vi "Configure Acquisition.vi"(0 "device session in":refnum<class "Device Session.lvclass">, 1 "pretrigger samples":u64, 2 "number of records is finite (T)":bool=TRUE, 5 "number of records":u64=1, 7 "number of samples":u64=1000, 9 "channels to store":u32[](array[numeric]), 11 "error in":errorcluster, 12 "additional configuration":T3={"record padding (samples)"=0, "require finite records to fit in memory"=TRUE, "timestamps per record"=1, "status fifo depth (records)"=10000}, 13 "Chan#":T2=enum."1") -> (4 "device session out":refnum<class "Device Session.lvclass">, 6 "actual channels stored":bool[](array[boolean]), 8 "TrigCount":u32[](array[numeric]), 10 "TrigCfg Array":T1(array[cluster]), 15 "error out":errorcluster)   [LabVIEW 2021, in "Device Session.lvclass"]
doc: "Configures the acquisition. You can specify which channels to acquire from, how many records to acquire, and how many samples to acquire. You must run this VI before running the <B>Initiate</B> VI.\n\n<B>Input Parameters</B>\n\n<B>device session in</B> is a reference to the Device Session object, which contains a session to each instrument design library used in this sample project. This parameter is obtained from the 'Open Session' VI.\n\n<B>number of records is finite (T)</B> specifies whether to acquire a finite number of records, or to acquire records continuously.\n\n<B>pretrigger samples</B> specifies, for every record, the minimum number of samples that must be stored from the time period immediately before the Reference Trigger occurred.\n\n<B>number of records</B> specifies the number of records to acquire. The default value is 1.\n\n<B>number of samples</B> specifies the number of samples to acquire. The default value is 1000.\n\n<B>channels to store</B> specifies the channels to store in memory. By default, only the channels configured using the 'Configure Channel' VI are stored.\n\n<B>additional configuration</B> specifies additional advanced configurations.\n\n<B>additional configuration.record padding (samples)</B> specifies additional padding to allocate for a record. This parameter can be useful in combination with adjusting the Reference Trigger position. The default value is 0.\n\n<B>additional configuration.require finite records to fit in memory</B> specifies that the requested number of records and samples must fit into memory for finite acquisitions. This parameter ensures that requested data cannot be overwritten for finite acquisitions. The default is TRUE.\n\n<B>additional configuration.timestamps per record</B> specifies the number of timestamp values the FPGA captures for each record. This value must match the number of timestamps per record provided to the Write VI of the Multirecord Acquisition FPGA library. The default value is 0.\n\n<B>additional configuration.status fifo depth (records)</B> Sets the depth of the record status DMA FIFO. The Status FIFO reports information about the current state of the acquisition to the host.\nEnsure that the Status FIFO is deep enough for the rate at which the host consumes this FIFO. If the Status FIFO is full, memory writes are delayed. Eventually, this can cause the Write FIFO to fill up and overflow. The host consumes the entire Status FIFO each time you fetch a record or query acquisition status. The value is specified in units of records. The default value is 10,000 records.\n\n<B>error in</B> describes error conditions that occur before this node runs. This input provides standard 'error in' functionality.\n\n<B>Output Parameters</B>\n\n<B>device session out</B> passes a reference to the session to the next VI.\n\n<B>actual channels stored</B> returns the number of channels stored as a power of two.\n\n<B>error out</B> contains error information. This output provides standard 'error out' functionality."
uses:
  Device Session.lvclass
  <instrlib>/_niInstr/Multirecord Acquisition/Interface/v1/Host/Public/Additional Acquisition Configuration.ctl
  Enums/Channel Numbers.ctl
  Device Session.lvclass/Device Session.ctl
  <vilib>/Utility/error.llb/Error Cluster From Error Code.vi
  <vilib>/rvi/errors/niLvFpgaAdjustHostInterfaceError.vi
  <vilib>/rvi/interface/nirviReadWriteControl/nirviReadWriteControl.xnode
  FPGA Refnum.ctl
  <instrlib>/_niInstr/Multirecord Acquisition/Interface/v1/Host/niInstr Multirecord Acquisition v1 Host.lvclass
  <vilib>/rvi/interface/Simulation/niFpgaSimulationCallBeginRW.vi
  NiFpgaLv.dll
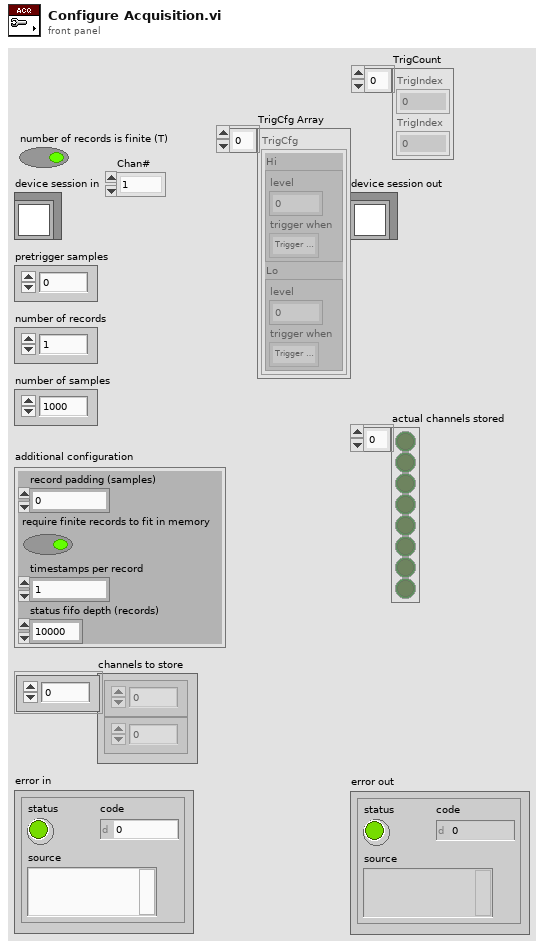
[diagram p1: front panel]
types:
  T1 = cluster{"Hi":cluster{"level":fxp<+/-,18,5>, "trigger when":enum8{"Trigger Above", "Trigger Below"}}, "Lo":cluster{"level":fxp<+/-,18,5>, "trigger when":enum8{"Trigger Above", "Trigger Below"}}}[]
  T2 = typedef "Channel Numbers.ctl" = enum16{"0", "1", "2", "3", "4", "5", "6", "7"}
  T3 = typedef "niInstr Multirecord Acquisition v1 Host.lvclass/Additional Acquisition Configuration.ctl" = cluster{"record padding (samples)":u64, "require finite records to fit in memory":bool, "timestamps per record":u32, "status fifo depth (records)":u32}
  T4 = typedef "Device Session.lvclass/Device Session Object.ctl" = cluster{"fpga reference":T5, "reg bus":refnum<class "niInstr FIFO Register Bus v1 Host.lvclass">, "subsystem map":refnum<class "niInstr Subsystem Map v1 Host.lvclass">, "cal data":refnum<class "niHSAI Cal Data v1 Host.lvclass">, "config":refnum<class "niHSAI Group A Config v1 Host.lvclass">, "acquisition 0":refnum<class "niInstr Multirecord Acquisition v1 Host.lvclass">, "acquisition 1":refnum<class "niInstr Multirecord Acquisition v1 Host.lvclass">, "acquisition 2":refnum<class "niInstr Multirecord Acquisition v1 Host.lvclass">, "acquisition 3":refnum<class "niInstr Multirecord Acquisition v1 Host.lvclass">, "acquisition 4":refnum<class "niInstr Multirecord Acquisition v1 Host.lvclass">, "acquisition 5":refnum<class "niInstr Multirecord Acquisition v1 Host.lvclass">, "acquisition 6":refnum<class "niInstr Multirecord Acquisition v1 Host.lvclass">, "acquisition 7":refnum<class "niInstr Multirecord Acquisition v1 Host.lvclass">, "number of selected acq channels":u8, "selected acq channels":bool[], "number of channels":u32, "configured channels":bool[], "acq configuration":cluster{"number of samples":u64, "number of records":u64, "pretrigger samples":u64}, "actual channel configuration":T6[], "sample clock rate (Hz)":dbl, "scaling coefficients":T10[]}
  T5 = typedef "Device Session.lvclass/FPGA Refnum.ctl" = refnum<k20>
  T6 = typedef "niHSAI Types v1 Host.lvlib/Channel Configuration.ctl" = cluster{"channel":u32, "coupling":T7, "impedance":T8, "bandwidth":T9, "vertical range":dbl, "vertical offset":dbl}
  T7 = typedef "niHSAI Types v1 Host.lvlib/Coupling.ctl" = enum8{"Default", "DC", "AC"}
  T8 = typedef "niHSAI Types v1 Host.lvlib/Impedance.ctl" = enum8{"Default", "1 mega ohm", "50 ohm"}
  T9 = typedef "niHSAI Types v1 Host.lvlib/Bandwidth.ctl" = enum8{"Default", "Full Bandwidth", "Anti-alias Filter", "150 MHz"}
  T10 = typedef "niInstr Multirecord Acquisition v1 Host.lvclass/Scaling Coefficient.ctl" = cluster{"gain":dbl, "offset":dbl}
  T11 = cluster{"Hi":cluster{"level":fxp<+/-,18,5>, "trigger when":enum8{"Trigger Above", "Trigger Below"}}, "Lo":cluster{"level":fxp<+/-,18,5>, "trigger when":enum8{"Trigger Above", "Trigger Below"}}}
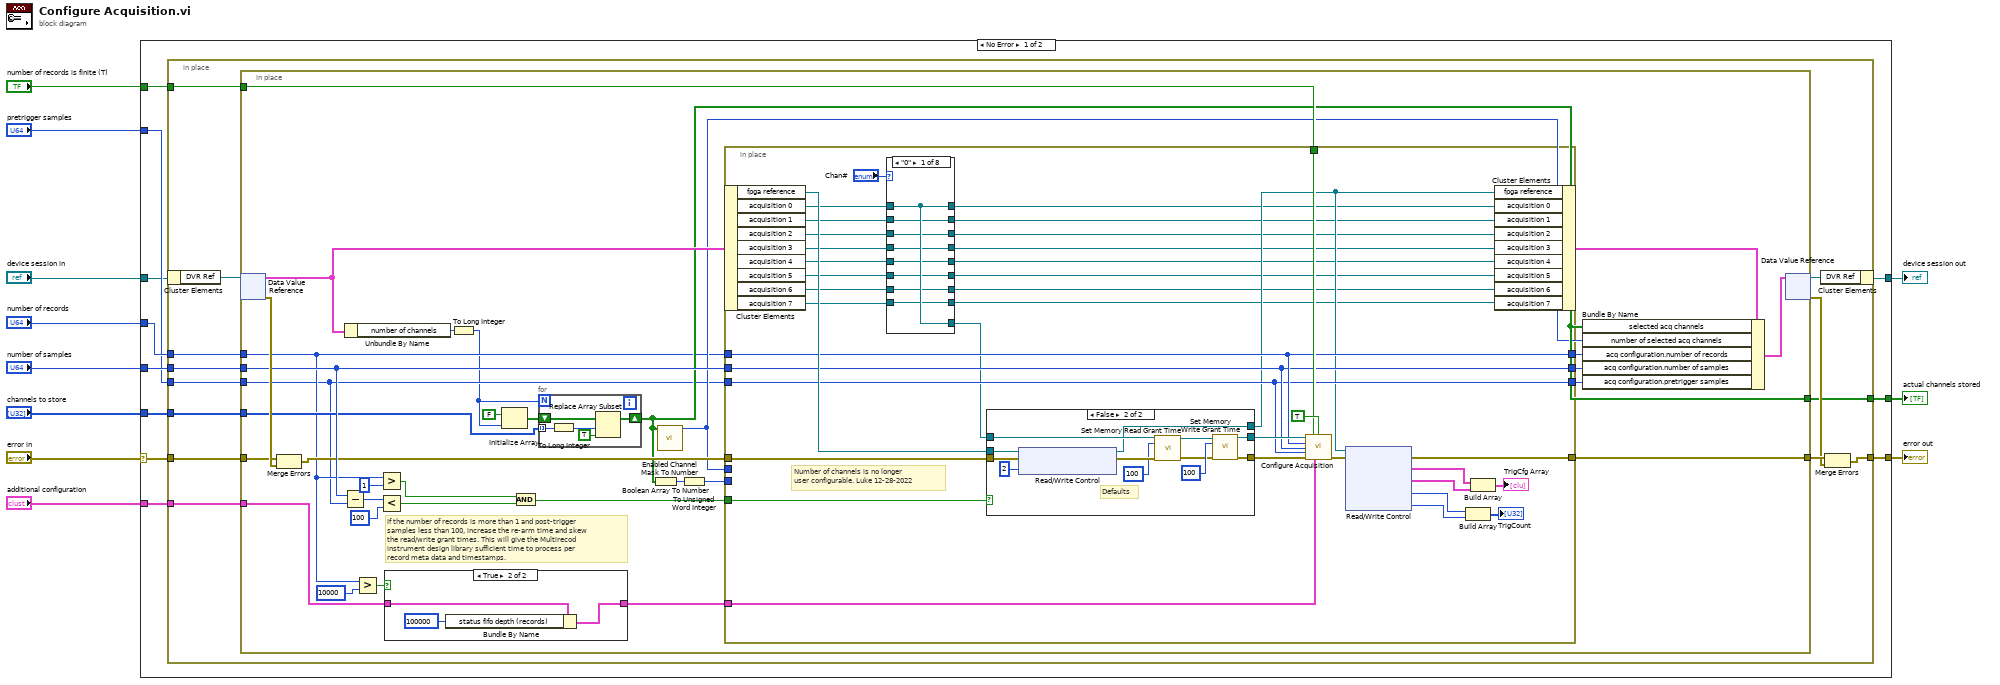
[diagram p0: block diagram]
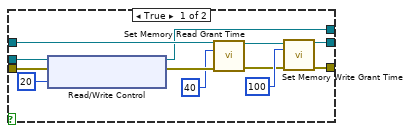
[diagram p9: hidden frame]
diagram:
  n1 = case shown="No Error" "error in" {
    selector: "error in" -> [w22 w205]
    tunnel: [w14 w205] -> w10
    tunnel: "device session in" -> [w12 w204]
    tunnel: [w13 w204] -> w8
    tunnel: "number of records" -> [w21 _]
    tunnel: "number of samples" -> [w20 _]
    tunnel: "channels to store" -> [w19 _]
    tunnel: [w18 _] -> w4
    tunnel: "pretrigger samples" -> [w17 _]
    tunnel: "additional configuration" -> [w16 _]
    tunnel: "number of records is finite (T)" -> [w15 _]
    frame No Error {
      n2 = in-place {
        in-place-border: w22 -> [w35]
        in-place-border: w21 -> [w34]
        in-place-border: w20 -> [w33]
        in-place-border: w19 -> [w30]
        in-place-border: [w29] -> w18
        in-place-border: w17 -> [w28]
        in-place-border: w16 -> [w27]
        in-place-border: w15 -> [w26]
        in-place-border: [w25] -> w14
        n3 = in-place-cluster #1(w12) -> ("DVR Ref"=w24:refnum<data-value>)
        n4 = in-place {
          in-place-border: w35 -> [w63]
          in-place-border: [w66] -> w32
          in-place-border: w34 -> [w38]
          in-place-border: w33 -> [w50]
          in-place-border: w30 -> [w39]
          in-place-border: [w44] -> w29
          in-place-border: w28 -> [w37]
          in-place-border: w27 -> [w48]
          in-place-border: w26 -> [w60]
          # "If the number of records is more than 1 and post-trigger samples less than 100, increase the re-arm time and skew the read/write grant times. This will give the Multirecod instrument design library sufficient time to process per record meta data and timestamps."
          n5 = in-place-dvr #2(w24) -> (w46:T4, w67:errorcluster)
          n6 = Merge Errors(w63, w67) -> (w49:errorcluster)
          n7 = Subtract(x=w50, y=w37) -> (x-y=w58:u64)
          n8 = Unbundle By Name(w46) -> ("number of channels"=w59:u32)
          n9 = Greater?(x=w38, y=u64 10000) -> (0:w51:bool)
          n10 = Greater?(x=w38, y=u64 1) -> (0:w55:bool)
          n11 = Less?(x=w58, y=u64 100) -> (x < y?=w54:bool)
          n12 = case shown="True" w51 {
            tunnel: w48 -> [w195 w198]
            tunnel: [w195 w196] -> w47
            frame False {
            }
            frame True {
              n13 = Bundle By Name(cluster=w198, "status fifo depth (records)"=u32 100000) -> (w196:T3)
            }
          }
          n14 = To Long Integer(number=w59) -> (32bit integer=w36:i32)
          n15 = Initialize Array(FALSE, w36) -> (w61:bool[])
          n16 = And(x=w55, y=w54) -> (x .and. y?=w53:bool)
          n17 = for {
            N: w36 -> [_]
            tunnel: w39 -> [w200] mode=indexing
            shift-right: [w202] -> w44
            shift-left: w61 -> [w201]
            n18 = To Long Integer(number=w200) -> (32bit integer=w199:i32)
            n19 = Replace Array Subset(array=w201, new element=TRUE ("new element/subarray"), index=w199) -> (w202:bool[])
          }
          n20 = Boolean Array To Number(Boolean array=w44) -> (number=w65:u32)
          n21 = call "Enabled Channel Mask To Number.vi"("selected acquisition channels to store"=w44) -> ("number of selected channels"=w43:u8)  [unwired: 14 in]
          n22 = To Unsigned Word Integer(number=w65) -> (unsigned 16bit integer=w64:u16)
          n23 = in-place {
            in-place-border: [w94] -> w66
            in-place-border: w64 -> [_]
            in-place-border: w60 -> [w105]
            in-place-border: w53 -> [w102]
            in-place-border: w37 -> [w96]
            in-place-border: w50 -> [w97]
            in-place-border: w49 -> [w101]
            in-place-border: w38 -> [w98]
            in-place-border: w43 -> [_]
            in-place-border: w47 -> [w100]
            in-place-border: [w98] -> w42
            in-place-border: [w97] -> w41
            in-place-border: [w96] -> w40
            # "Number of channels is no longer\nuser configurable. Luke 12-28-2022"
            n24 = in-place-cluster #3(w46) -> ("fpga reference"=w99:T5, "acquisition 0"=w91:refnum<class "niInstr Multirecord Acquisition v1 Host.lvclass">, "acquisition 1"=w90:refnum<class "niInstr Multirecord Acquisition v1 Host.lvclass">, "acquisition 2"=w88:refnum<class "niInstr Multirecord Acquisition v1 Host.lvclass">, "acquisition 3"=w87:refnum<class "niInstr Multirecord Acquisition v1 Host.lvclass">, "acquisition 4"=w86:refnum<class "niInstr Multirecord Acquisition v1 Host.lvclass">, "acquisition 5"=w85:refnum<class "niInstr Multirecord Acquisition v1 Host.lvclass">, "acquisition 6"=w84:refnum<class "niInstr Multirecord Acquisition v1 Host.lvclass">, "acquisition 7"=w83:refnum<class "niInstr Multirecord Acquisition v1 Host.lvclass">)
            n25 = case shown="\"0\"" "Chan#" {
              tunnel: w91 -> [w114 w121 w129 w137 w145 w153 w161 w169]
              tunnel: w90 -> [w113 w122 w128 w136 w144 w152 w160 w168]
              tunnel: [w114 w122 w130 w138 w146 w154 w162 w170] -> w89
              tunnel: w88 -> [w112 w120 w130 w135 w143 w151 w159 w167]
              tunnel: w87 -> [w111 w119 w127 w138 w142 w150 w158 w166]
              tunnel: w86 -> [w110 w118 w126 w134 w146 w149 w157 w165]
              tunnel: w85 -> [w109 w117 w125 w133 w141 w154 w156 w164]
              tunnel: w84 -> [w108 w116 w124 w132 w140 w148 w162 w163]
              tunnel: w83 -> [w107 w115 w123 w131 w139 w147 w155 w170]
              tunnel: [w114 w121 w129 w137 w145 w153 w161 w169] -> w82
              tunnel: [w113 w122 w128 w136 w144 w152 w160 w168] -> w81
              tunnel: [w112 w120 w130 w135 w143 w151 w159 w167] -> w80
              tunnel: [w111 w119 w127 w138 w142 w150 w158 w166] -> w79
              tunnel: [w110 w118 w126 w134 w146 w149 w157 w165] -> w78
              tunnel: [w109 w117 w125 w133 w141 w154 w156 w164] -> w77
              tunnel: [w108 w116 w124 w132 w140 w148 w162 w163] -> w76
              tunnel: [w107 w115 w123 w131 w139 w147 w155 w170] -> w75
              frame "0" {
              }
              frame "1" {
              }
              frame "2" {
              }
              frame "3" {
              }
              frame "4" {
              }
              frame "5" {
              }
              frame "6" {
              }
              frame "7" {
              }
            }
            n26 = case shown="False" w102 {
              tunnel: w89 -> [w176 w188]
              tunnel: w99 -> [w177 w189]
              tunnel: w101 -> [w175 w187]
              tunnel: [w174 w186] -> w104
              tunnel: [w173 w185] -> w103
              tunnel: [w171 w183] -> w93
              frame True {
                n27 = xnode "Read/Write Control"("FPGA VI Reference In"=w177, "error in"=w175, "trigger.rearm delay"=u16 20 ("trigger.rearm time")) -> ("FPGA VI Reference Out"=w171:T5, "error out"=w182:errorcluster)
                n28 = call-dynamic "Set Memory Read Grant Time.vi"("session in"=w176, "grant time (clocks)"=u32 40, "error in"=w182) -> ("session out"=w178:refnum<class "niInstr Multirecord Acquisition v1 Host.lvclass">, "error out"=w179:errorcluster)  [unwired: 11 in]
                n29 = call-dynamic "Set Memory Write Grant Time.vi"("session in"=w178, "grant time (clocks)"=u32 100, "error in"=w179) -> ("session out"=w173:refnum<class "niInstr Multirecord Acquisition v1 Host.lvclass">, "error out"=w174:errorcluster)  [unwired: 11 in]
              }
              frame False {
                # "Defaults"
                n30 = xnode "Read/Write Control"("FPGA VI Reference In"=w189, "error in"=w187, "trigger.rearm delay"=u16 2 ("trigger.rearm time")) -> ("FPGA VI Reference Out"=w183:T5, "error out"=w194:errorcluster)
                n31 = call-dynamic "Set Memory Read Grant Time.vi"("session in"=w188, "grant time (clocks)"=u32 100, "error in"=w194) -> ("session out"=w190:refnum<class "niInstr Multirecord Acquisition v1 Host.lvclass">, "error out"=w191:errorcluster)  [unwired: 11 in]
                n32 = call-dynamic "Set Memory Write Grant Time.vi"("session in"=w190, "grant time (clocks)"=u32 100, "error in"=w191) -> ("session out"=w185:refnum<class "niInstr Multirecord Acquisition v1 Host.lvclass">, "error out"=w186:errorcluster)  [unwired: 11 in]
              }
            }
            n33 = call-dynamic "Configure Acquisition.vi"("session in"=w103, "number of records is finite"=w105, "number of samples is finite"=TRUE, "number of records"=w98, "number of samples"=w97, "pretrigger samples"=w96, "error in"=w104, "additional acquisition configuration"=w100) -> ("error out"=w95:errorcluster)  [unwired: 5 in, 2 out]
            n34 = xnode "Read/Write Control"("FPGA VI Reference In"=w93, "error in"=w95) -> ("error out"=w94:errorcluster, "TrigCfg 0"=w74:T11, "TrigCfg 1"=w73:T11, "TrigCount"=w71:u32, "TrigCount 2"=w70:u32)  [unwired: 1 out]
            n35 = Build Array(w71, w70) -> (→"TrigCount":u32[])
            n36 = Build Array(w74, w73) -> (→"TrigCfg Array":T1)
            n37 = in-place-cluster #3("fpga reference"=w93, "acquisition 0"=w82, "acquisition 1"=w81, "acquisition 2"=w80, "acquisition 3"=w79, "acquisition 4"=w78, "acquisition 5"=w77, "acquisition 6"=w76, "acquisition 7"=w75) -> (w45:T4)
          }
          n38 = Bundle By Name(cluster=w45, "selected acq channels"=w44, "number of selected acq channels"=w43, "acq configuration.number of records"=w42, "acq configuration.number of samples"=w41, "acq configuration.pretrigger samples"=w40) -> (w68:T4)
          n39 = in-place-dvr #2(w68) -> (w23:refnum<data-value>, w31:errorcluster)
        }
        n40 = in-place-cluster #1("DVR Ref"=w23) -> (w13:refnum<class "Device Session.lvclass">)
        n41 = Merge Errors(w32, w31) -> (w25:errorcluster)
      }
    }
    frame Error {
    }
  }
  "error out" <- w10
  "device session out" <- w8
  "actual channels stored" <- w4
